vi "log_message.vi"(8 "error in (no error)":errorcluster, 9 "message":string, 11 "Logger in":refnum<class "WebSocket Queue Logger.lvclass">) -> (0 "error out":errorcluster, 3 "Logger out":refnum<class "WebSocket Queue Logger.lvclass">)   [LabVIEW 2019, in "WebSocket Server Toolkit.lvlib" / "WebSocket Queue Logger.lvclass"]
uses:
  WebSocket Queue Logger.lvclass
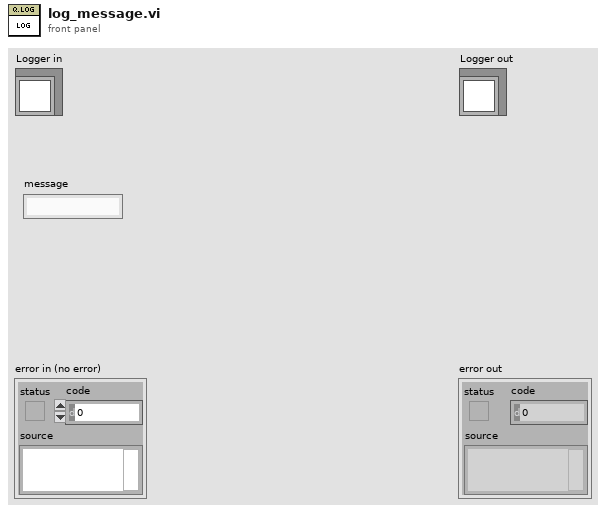
[diagram p1: front panel]
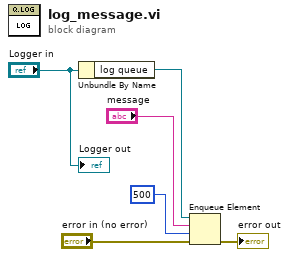
[diagram p0: block diagram]
diagram:
  n1 = Unbundle By Name("Logger in") -> ("log queue"=w5:refnum<queue>)
  n2 = Enqueue Element(queue=w5, element="message", timeout in ms (-1)=500, error in (no error)="error in (no error)") -> (error out=→"error out":errorcluster)  [unwired: 2 out]
  "Logger out" <- "Logger in"
